vi "Test_eeprom_read.vi"() -> ()   [LabVIEW 2019]
panel:
  out "Value response 2":u32
  out "Key response 2":u32
  out "unsigned byte array 2":u8[](array[numeric])
  out "unsigned byte array":u8[](array[numeric])
  out "Value response":u32
  out "Key response":u32
  in  "eeprom address":u32
  in  "Address":u8
  in  "COM Port for serial\nconnection. Check device\nmanager.":string
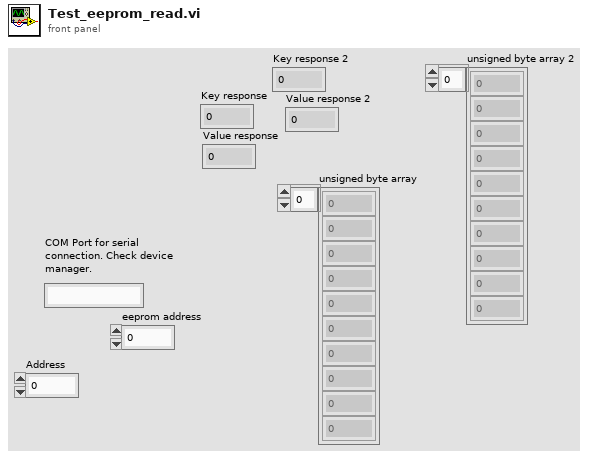
[diagram p1: front panel]
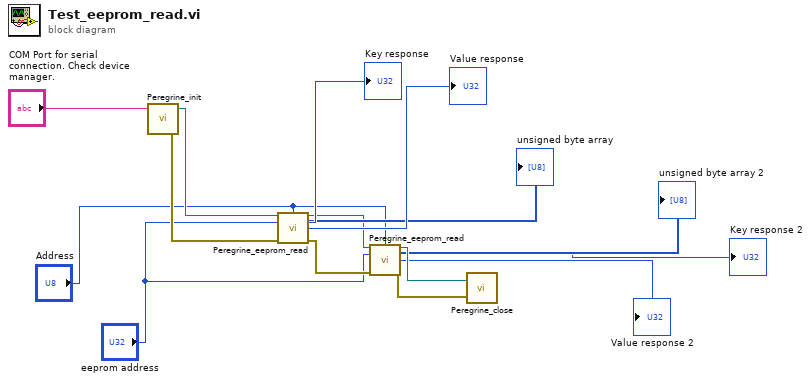
[diagram p0: block diagram]
diagram:
  n1 = call "Peregrine_init.vi"("COM Port for serial\nconnection. Check device\nmanager."="COM Port for serial\nconnection. Check device\nmanager.") -> ("error out"=w13:errorcluster, "Handle out"=w14:refnum<visa-resource-name>)  [unwired: 3 in]
  n2 = call "Peregrine_eeprom_read.vi"("Handle in"=w14, "Address"="Address", "eeprom address"="eeprom address", "error"=w13) -> ("unsigned byte array"=→"unsigned byte array":u8[], "Handle out"=w9:refnum<visa-resource-name>, "Key response"=→"Key response":u32, "Value response"=→"Value response":u32, "error out"=w8:errorcluster)  [unwired: 7 in]
  n3 = call "Peregrine_eeprom_read.vi"("Handle in"=w9, "Address"="Address", "eeprom address"="eeprom address", "error"=w8) -> ("unsigned byte array"=→"unsigned byte array 2":u8[], "Handle out"=w7:refnum<visa-resource-name>, "Key response"=→"Key response 2":u32, "Value response"=→"Value response 2":u32, "error out"=w6:errorcluster)  [unwired: 7 in]
  n4 = call "Peregrine_close.vi"("error in (no error)"=w6, "Handle in"=w7) -> ()  [unwired: 1 in, 1 out]
